vi "Scheduler.vi"(11 "Name (\"\" to Use UUID)":string) -> ()   [LabVIEW 2025]
uses:
  supports/Waypoint.ctl
  d7dd9159-89a2-4514-95bd-649e26e943bd.vi
  <vilib>/numeric/Random Number (Range) I64.vi
  e4e6d57c-e643-45f7-bca7-d28f1c2b9474.vi
  49f21eb9-f673-4fa8-8715-351f05abaff7.vi
  0d6ab66a-5149-4c79-b89e-f55ee53f3b39.vi
  3f08c095-eb42-4770-a6b1-2c55b3203edd.vi
  cd06cb13-84a1-4604-9614-019e20008b86.vi
  f0e5e5ea-bc13-4fd2-839c-8ba34e31ea16.vi
  <userlib>/_NEVSTOP/Communicable State Machine(CSM)/AdvanceAPI/CSM - Revert Arguments-Safe String.vi
  <userlib>/_NEVSTOP/Communicable State Machine(CSM)/AdvanceAPI/CSM - Make String Arguments Safe.vi
  <userlib>/_NEVSTOP/Communicable State Machine(CSM)/AdvanceAPI/CSM - Break Down Multiple States String.vi
  <userlib>/_NEVSTOP/Communicable State Machine(CSM)/AdvanceAPI/CSM - Compact Multiple States.vi
  <vilib>/numeric/sub_Random U32.vi
  <userlib>/_NEVSTOP/Communicable State Machine(CSM)/AdvanceAPI/CSM - Keywords.vi
  <userlib>/_NEVSTOP/Communicable State Machine(CSM)/_Shared/Trim Single-line Text.vi
  <userlib>/_NEVSTOP/Communicable State Machine(CSM)/addons/MassData-Parameter/_support/FGV-MassData(lvlibp).vi
  <userlib>/_NEVSTOP/Communicable State Machine(CSM)/_Polymophic/Build Status Broadcast Message.vi
  <userlib>/_NEVSTOP/Communicable State Machine(CSM)/_Polymophic/Build Synchronous Message with Arguments.vi
  <userlib>/_NEVSTOP/Communicable State Machine(CSM)/Communicable State Machine.lvlib
panel:
  out "Error Occurred":errorcluster
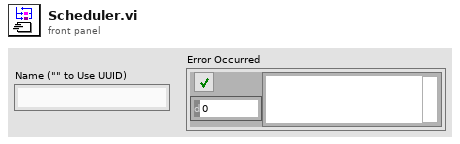
[diagram p1: front panel]
types:
  T1 = enum32{"Invalid", "Standard", "Closed", "Hidden", "Minimized", "Maximized"}
  T2 = enum32{"invalid app kind", "Development System", "Run Time System", "Student Edition", "Embedded LabVIEW", "Evaluation", "Custom"}
  T3 = typedef "Waypoint.ctl" = cluster{"x":i32, "y":i32}
  T4 = typedef "Communicable State Machine.lvlib/_CSM_Response Source Message.ctl" = cluster{"‘State":string, "’Arguments":string, "’Error":errorcluster}
  T5 = cluster{"Current VI Reference":refnum<vi>, "Close Panel on Exit?":bool}
  T6 = cluster{"Core":cluster{"Current VI Reference":refnum<vi>, "Close Panel on Exit?":bool}, "Level":i32, "Path":T3[], "Waypoint":T3, "Strike":i32, "Strikeout":i32, "Trial Count":i32}
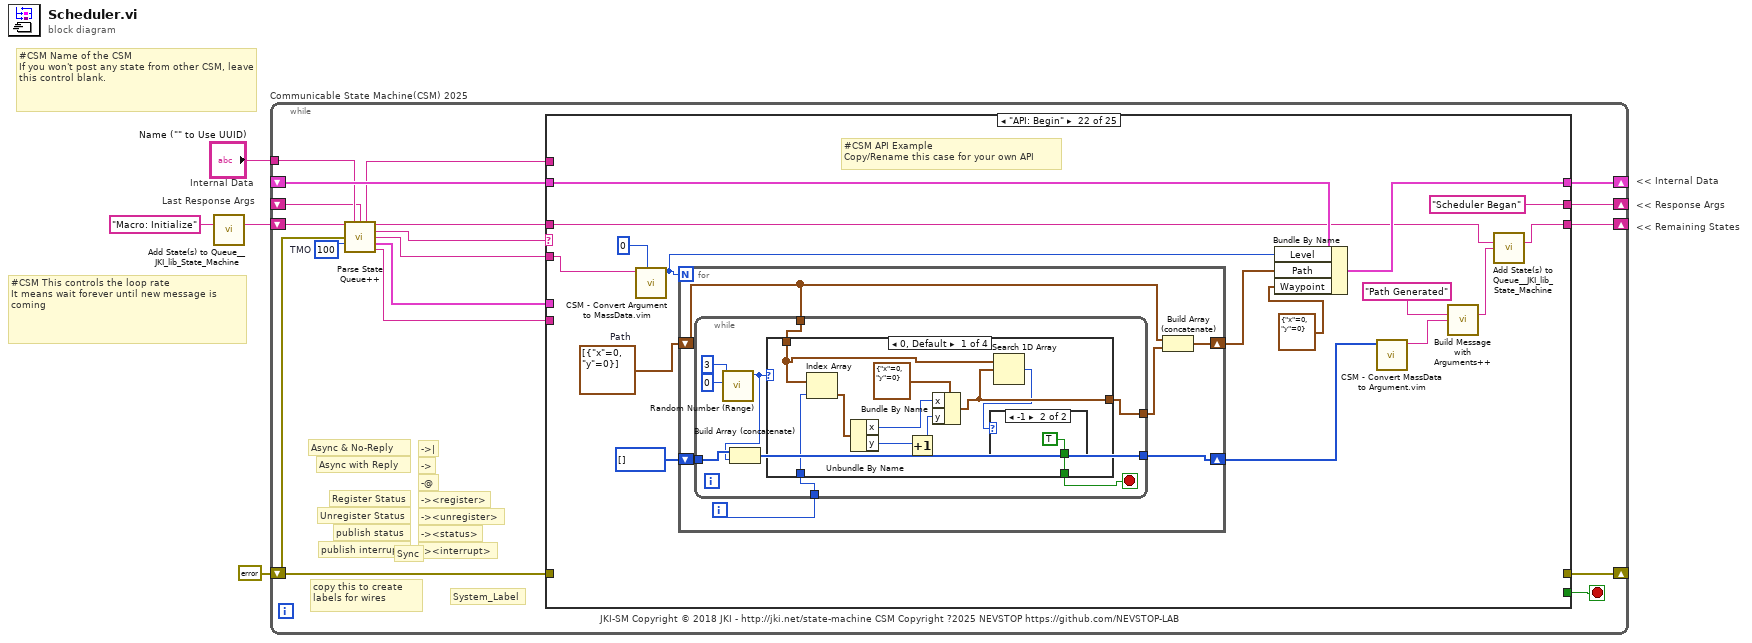
[diagram p0: block diagram]
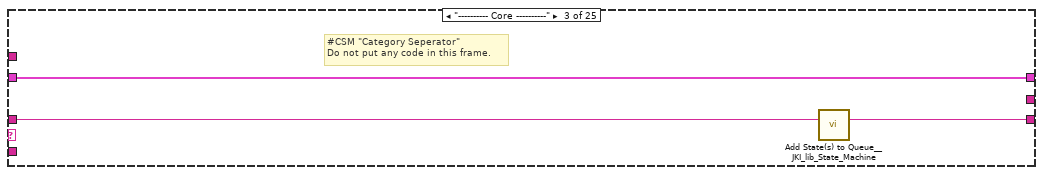
[diagram p4: hidden frame]
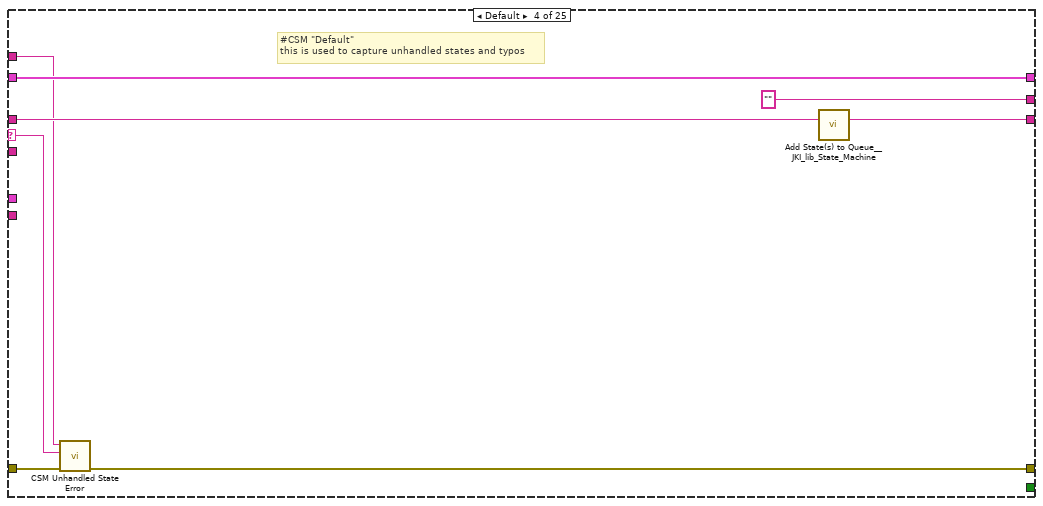
[diagram p5: hidden frame]
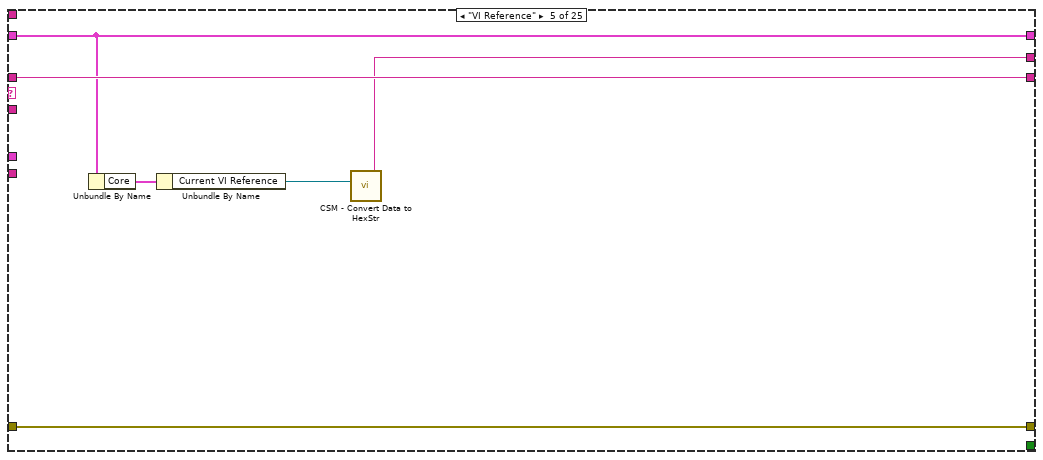
[diagram p6: hidden frame]
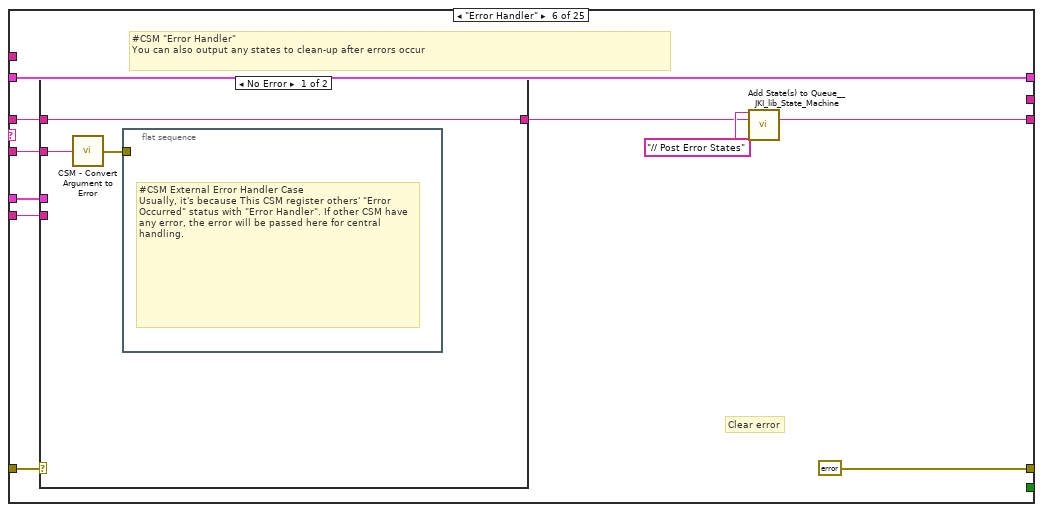
[diagram p7: hidden frame]
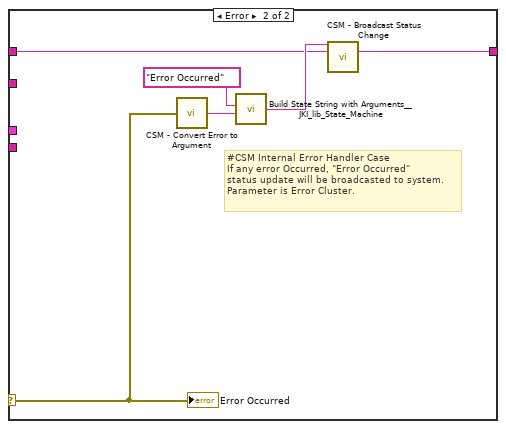
[diagram p8: hidden frame]
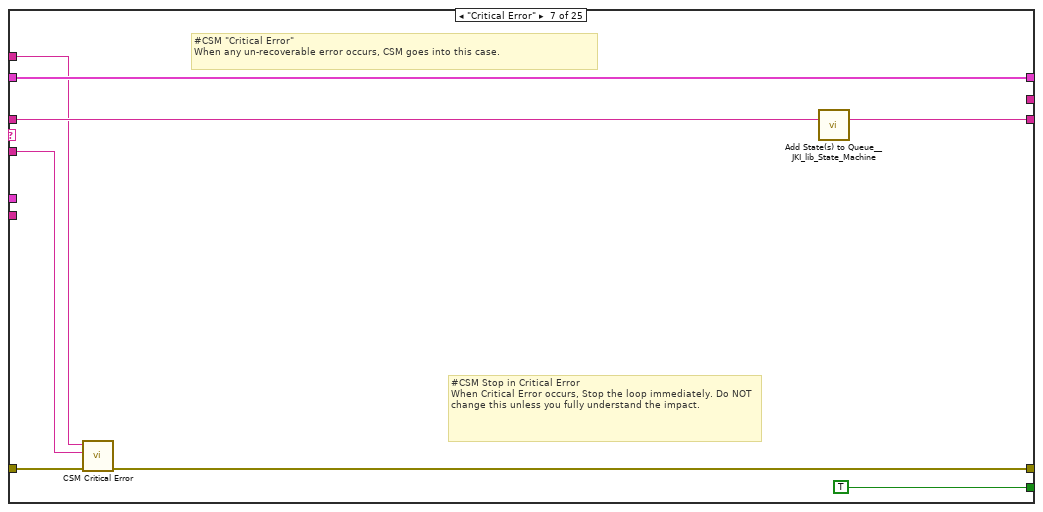
[diagram p9: hidden frame]
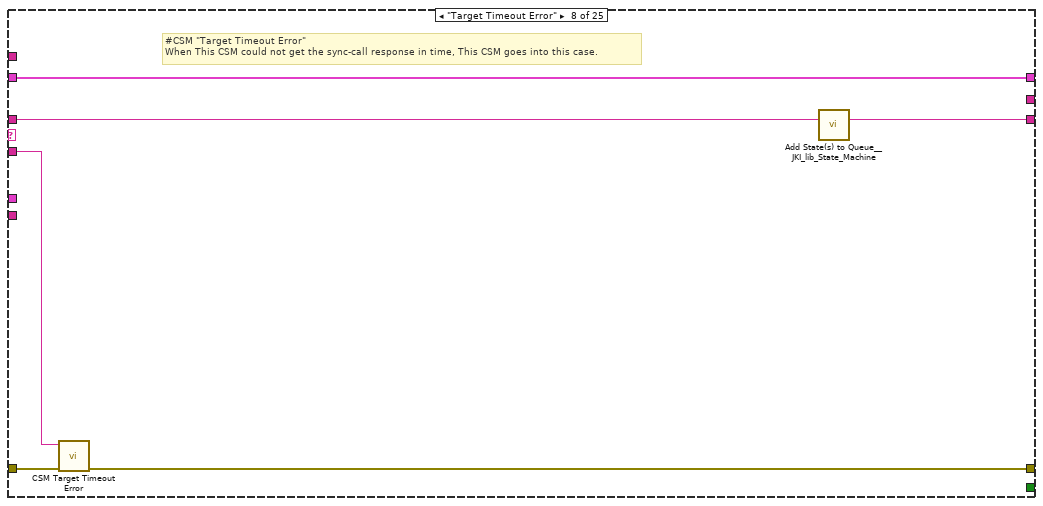
[diagram p10: hidden frame]
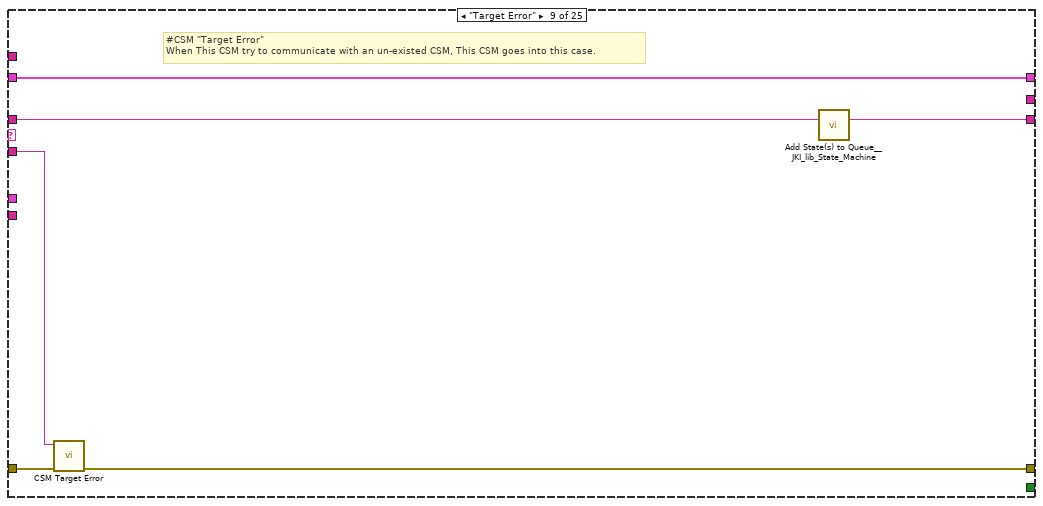
[diagram p11: hidden frame]
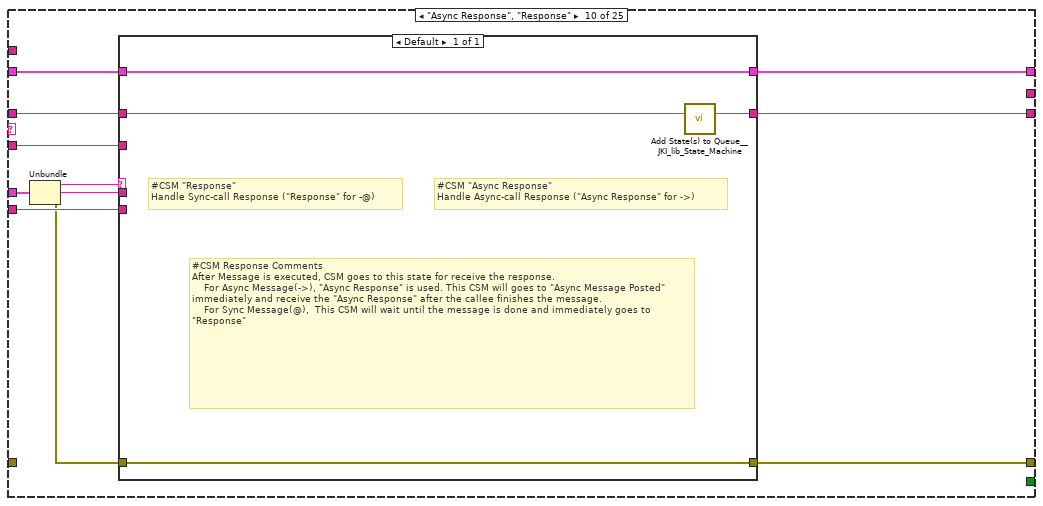
[diagram p12: hidden frame]
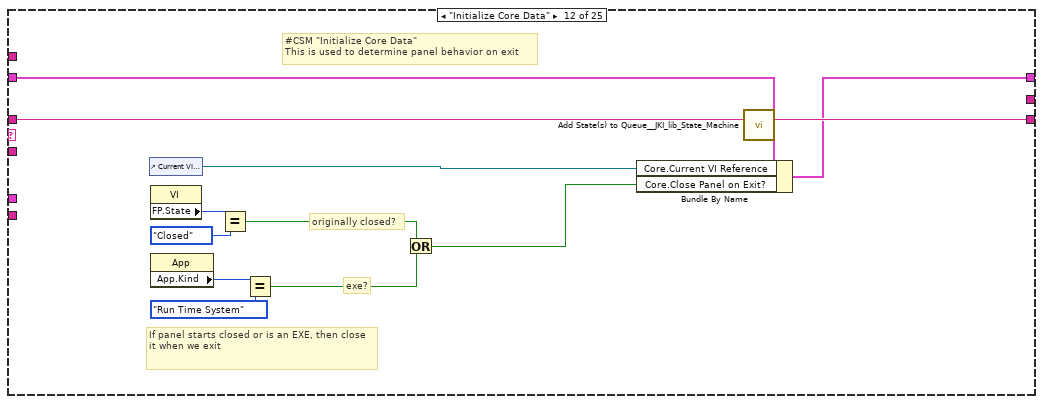
[diagram p14: hidden frame]
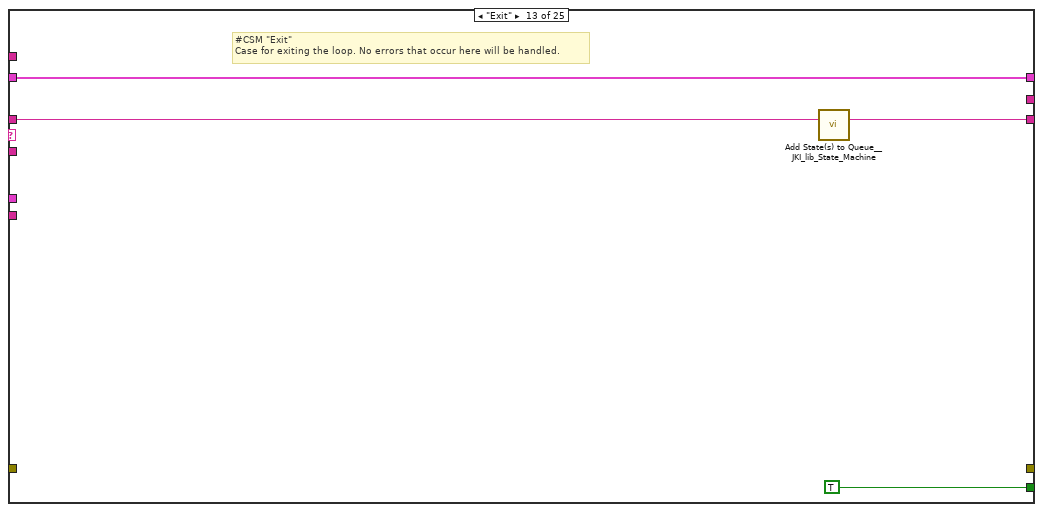
[diagram p15: hidden frame]
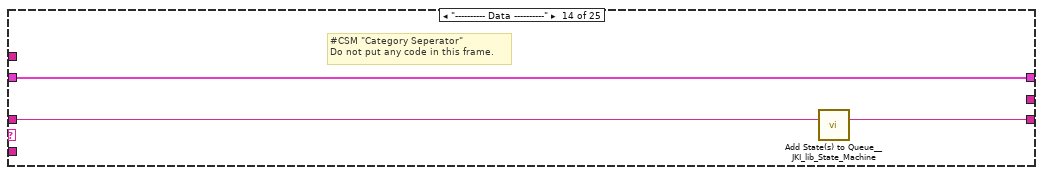
[diagram p16: hidden frame]
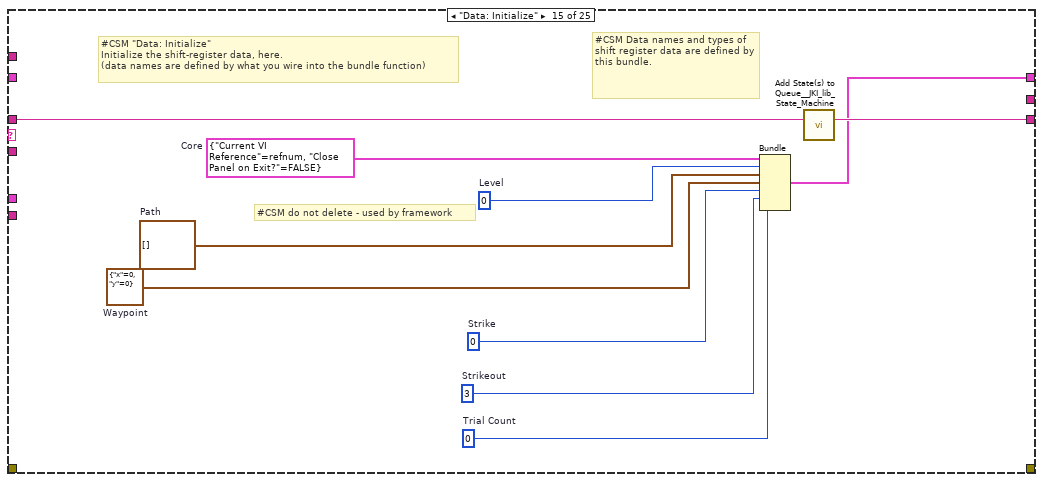
[diagram p17: hidden frame]
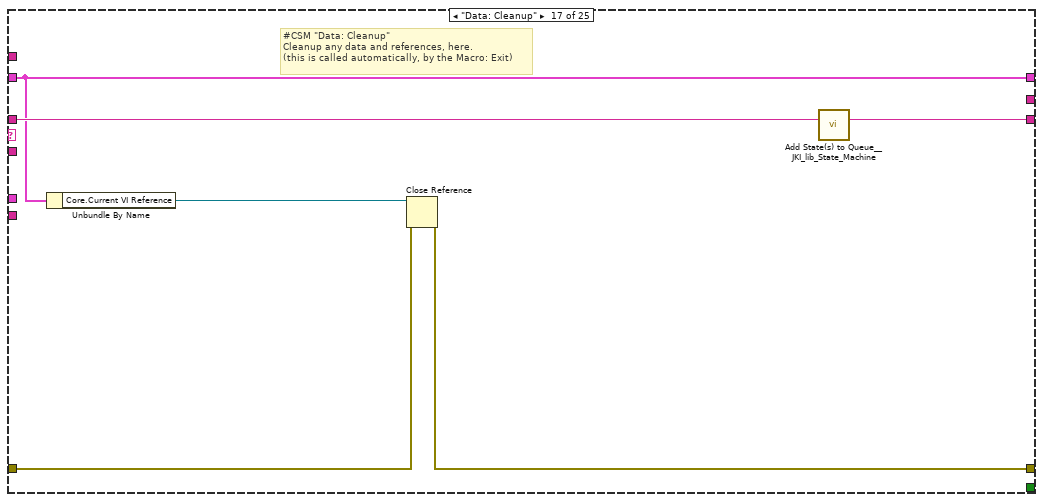
[diagram p19: hidden frame]
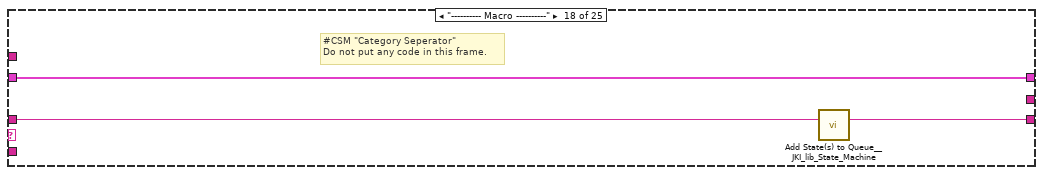
[diagram p20: hidden frame]
diagram:
  # "Last Response Args"
  # "Internal Data"
  # "#CSM Name of the CSM\nIf you won't post any state from other CSM, leave this control blank."
  # "#CSM This controls the loop rate\nIt means wait forever until new message is coming"
  # "<< Internal Data"
  # "<< Response Args"
  # "<< Remaining States"
  n1 = call <vilib>:"Add State(s) to Queue__JKI_lib_State_Machine.vi"("State(s) in (\"\")"="Macro: Initialize" ("Init State(\"Macro: Initialize\")")) -> ("States Out"=w1:string)  [unwired: 14 in]
  n2 = while "Communicable State Machine(CSM) 2025" {
    shift-right: [w16] -> _
    shift-left: _ -> [w15]
    shift-right: [w19] -> _
    shift-left: errorcluster {"status"=FALSE, "code"=0, "source"=""} ("error out") -> [w5]
    shift-right: [w18] -> _
    shift-left: w1 -> [w20]
    tunnel: "Name (\"\" to Use UUID)" -> [w12]
    shift-right: [w13] -> _
    shift-left: _ -> [w7]
    stop <- w17 stop-if-true
    w14 = 100  # TMO
    # "-><interrupt>"
    # "-><status>"
    # "-><unregister>"
    # "-><register>"
    # "-@"
    # "->"
    # "->|"
    # "publish interrupt"
    # "publish status"
    # "Unregister Status"
    # "Register Status"
    # "Sync"
    # "Async with Reply"
    # "Async & No-Reply"
    # "JKI-SM Copyright © 2018 JKI - http://jki.net/state-machine CSM Copyright ?2025 NEVSTOP https://github.com/NEVSTOP-LAB"
    # "copy this to create labels for wires"
    # "System_Label"
    n3 = call <userlib>:"Parse State Queue++.vi"("State Queue"=w20, "Name (\"\" to Use UUID)"=w12, "Response Arguments"=w7, "Previous Error"=w5, "Dequeue (1 ms)"=w14) -> ("Name Used"=w6:string, "Remaining States"=w21:string, "Current State"=w8:string, "Arguments"=w9:string, "Additional Information"=w10:T4, "Source CSM"=w11:string)  [unwired: 5 in]
    n4 = case shown="\"API: Begin\"" w8 {
      selector: w8 -> [_ _ _ w32 _ _ _ _ _ _ _ _ _ _ _ _ _ _ _ _ _ _ _ _ _]
      tunnel: w21 -> [w22 w25 w28 w36 w41 w46 w69 w75 w81 w91 w98 w110 w114 w117 w127 w129 w135 w138 w142 w148 w150 w158 w244 w371 w390]
      tunnel: w9 -> [_ _ _ _ _ w45 w65 w72 w78 w85 _ _ _ _ _ _ _ _ _ _ _ w164 w246 _ _]
      tunnel: w15 -> [w23 w24 w26 w34 w40 w51 w67 w73 w79 w89 w97 w104 w112 w115 _ w128 w130 w136 w140 w146 w149 w166 w245 w369 w383]
      tunnel: [_ _ _ w29 w42 errorcluster {"status"=FALSE, "code"=0, "source"=""} ("error out") w62 w70 w76 w92 _ _ _ _ _ _ w131 _ _ _ _ _ _ _ _] -> w19
      tunnel: w5 -> [_ _ _ w30 w42 w49 w63 w71 w77 _ _ _ _ _ _ _ w132 _ _ _ _ _ _ _ _]
      tunnel: [w22 w25 w27 w35 w41 w47 w68 w74 w80 w90 w98 w109 w113 w116 w126 w129 w134 w137 w141 w147 w150 w157 w240 w370 w389] -> w18
      tunnel: [_ _ _ _ _ _ TRUE _ _ _ _ _ TRUE _ _ _ _ _ _ _ _ _ _ _ _] -> w17
      tunnel: [w23 w24 w26 w34 w40 w51 w67 w73 w79 w88 w97 w108 w112 w115 w125 w128 w130 w136 w140 w146 w149 w165 w232 w369 w387] -> w16
      tunnel: w11 -> [_ _ _ _ _ w44 _ _ _ w86 _ _ _ _ _ _ _ _ _ _ _ _ _ _ _]
      tunnel: w10 -> [_ _ _ _ _ w43 _ _ _ w87 _ _ _ _ _ _ _ _ _ _ _ _ _ _ _]
      tunnel: [_ _ _ "" w37 _ _ _ _ _ _ _ _ _ _ _ _ _ _ _ _ "Scheduler Began" ("HEX String (0-9,A-F)") _ _ _] -> w13
      tunnel: w6 -> [_ _ _ w31 _ _ w64 _ _ _ _ _ _ _ _ _ _ _ _ _ _ _ _ _ _]
      frame "", "Idle" {
        # "#CSM \"Idle/Event Handler\"\nexecutes when the state queue is empty"
      }
      frame "CSM Documentation" {
        # "#CSM State Syntax\n\n// Comment line, all text to the right of “//” will be ignored\n// Local Message Example\nDoSth: DoA >> Arguments\n\n// Sync Call Example\nAPI: xxxx >> Arguments -@ TargetModule\n\n// Async Call Example\nAPI: xxxx >> Arguments -> TargetModule\n\n// Async Call without Reply Example\nAPI: xxxx >> Arguments ->| TargetModule\n\n// Broadcast normal status:\nStatus >> StatusArguments  -><status>\n\n// Broadcast Interrupt status:\nInterrupt >> StatusArguments  -><interrupt>\n\n// Register Source Module's status to Handler Module\nStatus@Source Module >> Handler Module@Handler Module -><register>\n\n// Unegister Source Module's status\nStatus@Source Module >> Handler Module -><unregister>"
        # "#CSM README FIRST\n\nCommunicable State Machine(CSM) is a LabVIEW application framework that builds upon JKI State Machine(JKISM). It follows the pattern of JKISM and extends the keywords to describe message communication between modules, including concepts such as Sync-Message, Async-Message, Subscription/Unsubscription of status - essential elements for creating reusable code modules. For more information, please visit the CSM wiki: https://nevstop-lab.github.io/CSM-Wiki/\n\nFor instructions on JKI State Machine, visit: \n    http://jki.net/state-machine/\nFor information about CSM, visit: \n    https://github.com/NEVSTOP-LAB"
        # "#CSM \"Documentation\"\nCase for holding CSM Documenation"
      }
      frame "---------- Core ----------" {
        # "#CSM \"Category Seperator\"\nDo not put any code in this frame."
        n5 = call <vilib>:"Add State(s) to Queue__JKI_lib_State_Machine.vi"("State(s) in (\"\")"=w28) -> ("States Out"=w27:string)  [unwired: 14 in]
      }
      frame Default {
        # "#CSM \"Default\"\nthis is used to capture unhandled states and typos"
        n6 = call <userlib>:"CSM Unhandled State Error.vi"("error in (no error)"=w30, "Undefined State"=w32, "CSM Name"=w31) -> ("error out"=w29:errorcluster)  [unwired: 8 in]
        n7 = call <vilib>:"Add State(s) to Queue__JKI_lib_State_Machine.vi"("State(s) in (\"\")"=w36) -> ("States Out"=w35:string)  [unwired: 14 in]
      }
      frame "VI Reference" {
        n8 = Unbundle By Name(w40) -> ("Core"=w39:T5)
        n9 = Unbundle By Name(w39) -> ("Current VI Reference"=w38:refnum<vi>)
        n10 = call <userlib>:"CSM - Convert Data to HexStr.vi"("Variant"=w38) -> ("HEX String (0-9,A-F)"=w37:string)  [unwired: 8 in]
      }
      frame "Error Handler" {
        # "#CSM \"Error Handler\"\nYou can also output any states to clean-up after errors occur"
        # "Clear error"
        n11 = case shown="No Error" w49 {
          selector: w49 -> [_ w56]
          tunnel: [w55 w58] -> w48
          tunnel: w46 -> [w55 w57]
          tunnel: w45 -> [w54 _]
          tunnel: w44 -> [_ _]
          tunnel: w43 -> [_ _]
          frame No Error {
            n12 = call <userlib>:"CSM - Convert Argument to Error.vi"("Argument"=w54) -> ("Error"=w53:errorcluster)  [unwired: 4 in]
            n13 = flat-sequence {
              tunnel: w53 -> [_]
              frame #0 {
                # "#CSM External Error Handler Case\nUsually, it's because This CSM register others' \"Error Occurred\" status with \"Error Handler\". If other CSM have any error, the error will be passed here for central handling."
              }
            }
          }
          frame Error {
            # "#CSM Internal Error Handler Case \nIf any error Occurred, \"Error Occurred\" \nstatus update will be broadcasted to system.\nParameter is Error Cluster."
            n14 = call <userlib>:"CSM - Convert Error to Argument.vi"("Error"=w56) -> ("Argument"=w60:string)  [unwired: 4 in]
            n15 = call <vilib>:"Build State String with Arguments__JKI_lib_State_Machine.vi"("Arguments (\"\")"=w60, "State"="Error Occurred" ("Status with Arguments")) -> ("State with Arguments"=w59:string)  [unwired: 4 in]
            n16 = call <userlib>:"CSM - Broadcast Status Change.vi"("Status With Arguments"=w59, "State Queue"=w57) -> ("Remaining States"=w58:string)  [unwired: 13 in]
            "Error Occurred" <- w56
          }
        }
        n17 = call <vilib>:"Add State(s) to Queue__JKI_lib_State_Machine.vi"("State(s) in Front (\"\")"="// Post Error States", "State(s) in (\"\")"=w48) -> ("States Out"=w47:string)  [unwired: 13 in]
      }
      frame "Critical Error" {
        # "#CSM \"Critical Error\"\nWhen any un-recoverable error occurs, CSM goes into this case."
        # "#CSM Stop in Critical Error\nWhen Critical Error occurs, Stop the loop immediately. Do NOT change this unless you fully understand the impact."
        n18 = call <userlib>:"CSM Critical Error.vi"("error in (no error)"=w63, "Arugments (As Reason)"=w65, "CSM Name"=w64) -> ("error out"=w62:errorcluster)  [unwired: 8 in]
        n19 = call <vilib>:"Add State(s) to Queue__JKI_lib_State_Machine.vi"("State(s) in (\"\")"=w69) -> ("States Out"=w68:string)  [unwired: 14 in]
      }
      frame "Target Timeout Error" {
        # "#CSM \"Target Timeout Error\"\nWhen This CSM could not get the sync-call response in time, This CSM goes into this case."
        n20 = call <userlib>:"CSM Target Timeout Error.vi"("error in (no error)"=w71, "Arguments (As CSM Name)"=w72) -> ("error out"=w70:errorcluster)  [unwired: 9 in]
        n21 = call <vilib>:"Add State(s) to Queue__JKI_lib_State_Machine.vi"("State(s) in (\"\")"=w75) -> ("States Out"=w74:string)  [unwired: 14 in]
      }
      frame "Target Error" {
        # "#CSM \"Target Error\"\nWhen This CSM try to communicate with an un-existed CSM, This CSM goes into this case."
        n22 = call <userlib>:"CSM Target Error.vi"("error in (no error)"=w77, "Arguments (As CSM Name)"=w78) -> ("error out"=w76:errorcluster)  [unwired: 9 in]
        n23 = call <vilib>:"Add State(s) to Queue__JKI_lib_State_Machine.vi"("State(s) in (\"\")"=w81) -> ("States Out"=w80:string)  [unwired: 14 in]
      }
      frame "Async Response", "Response" {
        n24 = Unbundle(w87) -> ("‘State"=w84:string, "’Arguments"=w83:string, "’Error"=w82:errorcluster)
        n25 = case shown="Default" w84 {
          tunnel: [w93] -> w90
          tunnel: w91 -> [w94]
          tunnel: [w96] -> w88
          tunnel: w89 -> [w96]
          tunnel: [w95] -> w92
          tunnel: w82 -> [w95]
          tunnel: w86 -> [_]
          tunnel: w85 -> [_]
          tunnel: w83 -> [_]
          frame Default {
            # "#CSM \"Async Response\"\nHandle Async-call Response (\"Async Response\" for ->)"
            # "#CSM \"Response\"\nHandle Sync-call Response (\"Response\" for -@)"
            # "#CSM Response Comments\nAfter Message is executed, CSM goes to this state for receive the response.\n    For Async Message(->), \"Async Response\" is used. This CSM will goes to \"Async Message Posted\" immediately and receive the \"Async Response\" after the callee finishes the message.\n    For Sync Message(@),  This CSM will wait until the message is done and immediately goes to \"Response\""
            n26 = call <vilib>:"Add State(s) to Queue__JKI_lib_State_Machine.vi"("State(s) in (\"\")"=w94) -> ("States Out"=w93:string)  [unwired: 14 in]
          }
        }
      }
      frame "Async Message Posted" {
        # "#CSM \"Async Message Posted\"\nAfter Async Message is posted (-> or ->| ), CSM goes to this state for post-action.\nYou can use Argument - State to tell which Async Message is called."
      }
      frame "Initialize Core Data" {
        # "#CSM \"Initialize Core Data\"\nThis is used to determine panel behavior on exit"
        # "originally closed?"
        # "exe?"
        # "If panel starts closed or is an EXE, then close it when we exit"
        n27 = control-ref of="Current VI Reference"() -> (w102:refnum<vi>)
        n28 = property class="VI"() -> ("FP.State"=w101:T1)  [unwired: 2 in, 2 out]
        n29 = property class="App"() -> ("App.Kind"=w107:T2)  [unwired: 2 in, 2 out]
        n30 = Equal?(x=w101, y=T1."Closed" ("Front Panel Window:State")) -> (x = y?=w99:bool)
        n31 = Equal?(x=w107, y=T2."Run Time System" ("Application:Kind")) -> (x = y?=w105:bool)
        n32 = Or(x=w99, y=w105) -> (x .or. y?=w103:bool)
        n33 = Bundle By Name(cluster=w104, "Core.Current VI Reference"=w102, "Core.Close Panel on Exit?"=w103) -> (w108:T6)
        n34 = call <vilib>:"Add State(s) to Queue__JKI_lib_State_Machine.vi"("State(s) in (\"\")"=w110) -> ("States Out"=w109:string)  [unwired: 14 in]
      }
      frame "Exit" {
        # "#CSM \"Exit\"\nCase for exiting the loop. No errors that occur here will be handled."
        n35 = call <vilib>:"Add State(s) to Queue__JKI_lib_State_Machine.vi"("State(s) in (\"\")"=w114) -> ("States Out"=w113:string)  [unwired: 14 in]
      }
      frame "---------- Data ----------" {
        # "#CSM \"Category Seperator\"\nDo not put any code in this frame."
        n36 = call <vilib>:"Add State(s) to Queue__JKI_lib_State_Machine.vi"("State(s) in (\"\")"=w117) -> ("States Out"=w116:string)  [unwired: 14 in]
      }
      frame "Data: Initialize" {
        w118 = 0  # Trial Count
        w119 = 3  # Strikeout
        w120 = 0  # Strike
        w121 = T3 {"x"=0, "y"=0}  # Waypoint
        w122 = T3[] []  # Path
        w123 = 0  # Level
        w124 = T5 {"Current VI Reference"=refnum, "Close Panel on Exit?"=FALSE}  # Core
        # "#CSM \"Data: Initialize\"\nInitialize the shift-register data, here.\n(data names are defined by what you wire into the bundle function)"
        # "#CSM do not delete - used by framework"
        # "#CSM Data names and types of shift register data are defined by this bundle."
        n37 = Bundle("Core"=w124, "Level"=w123, "Path"=w122, "Waypoint"=w121, "Strike"=w120, "Strikeout"=w119, "Trial Count"=w118) -> (w125:T6)  [unwired: 1 in]
        n38 = call <vilib>:"Add State(s) to Queue__JKI_lib_State_Machine.vi"("State(s) in (\"\")"=w127) -> ("States Out"=w126:string)  [unwired: 14 in]
      }
      frame "Data: Update Indicators" {
      }
      frame "Data: Cleanup" {
        # "#CSM \"Data: Cleanup\"\nCleanup any data and references, here.\n(this is called automatically, by the Macro: Exit)"
        n39 = Unbundle By Name(w130) -> ("Core.Current VI Reference"=w133:refnum<vi>)
        n40 = Close Reference(reference=w133, error in (no error)=w132) -> (error out=w131:errorcluster)
        n41 = call <vilib>:"Add State(s) to Queue__JKI_lib_State_Machine.vi"("State(s) in (\"\")"=w135) -> ("States Out"=w134:string)  [unwired: 14 in]
      }
      frame "---------- Macro ----------" {
        # "#CSM \"Category Seperator\"\nDo not put any code in this frame."
        n42 = call <vilib>:"Add State(s) to Queue__JKI_lib_State_Machine.vi"("State(s) in (\"\")"=w138) -> ("States Out"=w137:string)  [unwired: 14 in]
      }
      frame "Macro: Initialize" {
        # "#CSM \"Macro: Initialize\"\nInitialization Macro (This is called once, when the VI starts)"
        n43 = call <vilib>:"Add State(s) to Queue__JKI_lib_State_Machine.vi"("State(s) in Front (\"\")"="Initialize Core Data\nData: Initialize\nData: Update Indicators", "State(s) in (\"\")"=w142) -> ("States Out"=w141:string)  [unwired: 13 in]
      }
      frame "Macro: Exit" {
        # "#CSM \"Macro: Exit\"\nExit Macro (This is called once, when the VI exits)"
        n44 = call <vilib>:"Add State(s) to Queue__JKI_lib_State_Machine.vi"("State(s) in Front (\"\")"="//Exit Sub-Modules ", "State(s) at Back (\"\")"="Data: Cleanup\nExit") -> ("States Out"=w144:string)  [unwired: 13 in]
        n45 = call <vilib>:"Add State(s) to Queue__JKI_lib_State_Machine.vi"("State(s) in Front (\"\")"=w144, "State(s) in (\"\")"=w148) -> ("States Out"=w147:string)  [unwired: 13 in]
      }
      frame "---------- API ----------" {
        # "#CSM \"Category Seperator\"\nDo not put any code in this frame."
      }
      frame "API: Begin" {
        w162 = T3[] [{"x"=0, "y"=0}]  # Path
        # "#CSM API Example\nCopy/Rename this case for your own API"
        n46 = call "CSM - Convert Argument to MassData.vim"("Type"=0, "MassData Argument"=w164) -> ("Data"=w160:i32)  [unwired: 6 in, 1 out]
        n47 = for {
          N: w160 -> [_]
          shift-right: [w172] -> w154
          shift-left: w162 -> [w171]
          shift-right: [w167] -> w151
          shift-left: i64[] [] ("appended array") -> [w168]
          i -> [w170]
          n48 = while {
            tunnel: w171 -> [w179]
            tunnel: w170 -> [w178]
            tunnel: [w177] -> w169
            tunnel: w168 -> [w175]
            tunnel: [w174] -> w167
            stop <- w176 stop-if-true
            n49 = call-poly <vilib>:"Random Number (Range).vi"("lower bound (-100)"=i64 0, "upper bound (100)"=i64 3) -> ("number"=w173:i64)  [unwired: 9 in]
            n50 = Build Array (concatenate)(w175, w173) -> (w174:i64[])
            n51 = case shown="0, Default" w173 {
              tunnel: w179 -> [w188 w200 w211 w221]
              tunnel: w178 -> [w191 w203 w215 w227]
              tunnel: [w187 w199 w210 w220] -> w177
              tunnel: [w185 w197 w208 w218] -> w176
              frame 0, Default {
                n52 = Index Array(array=w188, index=w191) -> (element=w190:T3)
                n53 = Unbundle By Name(w190) -> ("x"=w184:i32, "y"=w183:i32)
                n54 = Increment(x=w183) -> (x+1=w182:i32)
                n55 = Bundle By Name(cluster=T3 {"x"=0, "y"=0} ("Waypoint"), "x"=w184, "y"=w182) -> (w187:T3)
                n56 = Search 1D Array(1D array=w188, element=w187) -> (index of element=w186:i32)  [unwired: 1 in]
                n57 = case shown="-1" w186 {
                  tunnel: [FALSE TRUE] -> w185
                  frame Default {
                  }
                  frame -1 {
                  }
                }
              }
              frame 1 {
                n58 = Index Array(array=w200, index=w203) -> (element=w202:T3)
                n59 = Unbundle By Name(w202) -> ("x"=w196:i32, "y"=w195:i32)
                n60 = Decrement(x=w195) -> (x-1=w194:i32)
                n61 = Bundle By Name(cluster=T3 {"x"=0, "y"=0} ("Waypoint"), "x"=w196, "y"=w194) -> (w199:T3)
                n62 = Search 1D Array(1D array=w200, element=w199) -> (index of element=w198:i32)  [unwired: 1 in]
                n63 = case shown="-1" w198 {
                  tunnel: [FALSE TRUE] -> w197
                  frame Default {
                  }
                  frame -1 {
                  }
                }
              }
              frame 2 {
                n64 = Index Array(array=w211, index=w215) -> (element=w214:T3)
                n65 = Unbundle By Name(w214) -> ("x"=w207:i32, "y"=w212:i32)
                n66 = Decrement(x=w207) -> (x-1=w206:i32)
                n67 = Bundle By Name(cluster=T3 {"x"=0, "y"=0} ("Waypoint"), "x"=w206, "y"=w212) -> (w210:T3)
                n68 = Search 1D Array(1D array=w211, element=w210) -> (index of element=w209:i32)  [unwired: 1 in]
                n69 = case shown="-1" w209 {
                  tunnel: [FALSE TRUE] -> w208
                  frame Default {
                  }
                  frame -1 {
                  }
                }
              }
              frame 3 {
                n70 = Index Array(array=w221, index=w227) -> (element=w226:T3)
                n71 = Unbundle By Name(w226) -> ("x"=w225:i32, "y"=w222:i32)
                n72 = Increment(x=w225) -> (x+1=w224:i32)
                n73 = Bundle By Name(cluster=T3 {"x"=0, "y"=0} ("Waypoint"), "x"=w224, "y"=w222) -> (w220:T3)
                n74 = Search 1D Array(1D array=w221, element=w220) -> (index of element=w219:i32)  [unwired: 1 in]
                n75 = case shown="-1" w219 {
                  tunnel: [FALSE TRUE] -> w218
                  frame Default {
                  }
                  frame -1 {
                  }
                }
              }
            }
          }
          n76 = Build Array (concatenate)(w171, w169) -> (w172:T3[])
        }
        n77 = Bundle By Name(cluster=w166, "Level"=w160, "Path"=w154, "Waypoint"=T3 {"x"=0, "y"=0}) -> (w165:T6)
        n78 = call "CSM - Convert MassData to Argument.vim"("Data"=w151) -> ("MassData Argument"=w153:string)  [unwired: 7 in, 1 out]
        n79 = call-poly <userlib>:"Build Message with Arguments++.vi"("State With Arguments"="Path Generated", "Arguments (\"\")"=w153) -> ("CSM Message String"=w156:string)  [unwired: 13 in]
        n80 = call <vilib>:"Add State(s) to Queue__JKI_lib_State_Machine.vi"("State(s) in (\"\")"=w158, "State(s) at Back (\"\")"=w156) -> ("States Out"=w157:string)  [unwired: 13 in]
      }
      frame "API: Check Waypoint" {
        # "#CSM API Example\nCopy/Rename this case for your own API"
        n81 = case shown="\"Gate Up\"" w246 {
          tunnel: w245 -> [w264 w277 w303 w329 w355]
          tunnel: [w264 w267 w293 w320 w346] -> w233
          tunnel: "Gate Scheduled" -> [_ w272 w297 w317 w349]
          tunnel: [" \"Error Handler\" " w273 w296 w323 w343] -> w242
          frame Default {
          }
          frame "Gate Up" {
            n82 = Unbundle By Name(w277) -> ("Waypoint.x"=w278:i32, "Waypoint.y"=w280:i32)
            n83 = Increment(x=w280) -> (x+1=w279:i32)
            n84 = Bundle By Name(cluster=w277, "Waypoint.x"=w278, "Waypoint.y"=w279) -> (w268:T6)
            n85 = Unbundle By Name(w268) -> ("Path"=w275:T3[], "Waypoint"=w276:T3, "Level"=w269:i32, "Strike"=w266:i32)
            n86 = Search 1D Array(1D array=w275, element=w276) -> (index of element=w274:i32)  [unwired: 1 in]
            n87 = case shown="Default" w274 {
              selector: w274 -> [w284 _]
              tunnel: [w285 w290] -> w270
              tunnel: w269 -> [w283 _]
              tunnel: w266 -> [w281 w289]
              tunnel: [w281 w288] -> w265
              frame Default {
                n88 = Equal?(x=w284, y=w283) -> (x = y?=w282:bool)
                n89 = case shown="False" w282 {
                  tunnel: [w286 w287] -> w285
                  frame False {
                    w286 = bool[] [FALSE, FALSE, FALSE, FALSE]  # Gate Condition
                  }
                  frame True {
                    w287 = bool[] [TRUE, FALSE, TRUE, TRUE]  # Gate Condition
                  }
                }
              }
              frame -1 {
                w290 = bool[] [TRUE, FALSE, TRUE, TRUE]  # Gate Condition
                n90 = Increment(x=w289) -> (x+1=w288:i32)
              }
            }
            n91 = Bundle By Name(cluster=w268, "Strike"=w265) -> (w267:T6)
            n92 = call "CSM - Convert MassData to Argument.vim"("Data"=w270) -> ("MassData Argument"=w271:string)  [unwired: 7 in, 1 out]
            n93 = call-poly <userlib>:"Build Message with Arguments++.vi"("State With Arguments"=w272, "Arguments (\"\")"=w271) -> ("CSM Message String"=w273:string)  [unwired: 13 in]
          }
          frame "Gate Down" {
            n94 = Unbundle By Name(w303) -> ("Waypoint.x"=w305:i32, "Waypoint.y"=w306:i32)
            n95 = Decrement(x=w306) -> (x-1=w304:i32)
            n96 = Bundle By Name(cluster=w303, "Waypoint.x"=w305, "Waypoint.y"=w304) -> (w294:T6)
            n97 = Unbundle By Name(w294) -> ("Path"=w301:T3[], "Waypoint"=w302:T3, "Level"=w295:i32, "Strike"=w291:i32)
            n98 = Search 1D Array(1D array=w301, element=w302) -> (index of element=w300:i32)  [unwired: 1 in]
            n99 = case shown="Default" w300 {
              selector: w300 -> [w310 _]
              tunnel: [w308 w316] -> w299
              tunnel: w295 -> [w311 _]
              tunnel: [w307 w315] -> w292
              tunnel: w291 -> [w307 w314]
              frame Default {
                n100 = Equal?(x=w310, y=w311) -> (x = y?=w309:bool)
                n101 = case shown="False" w309 {
                  tunnel: [w312 w313] -> w308
                  frame False {
                    w312 = bool[] [FALSE, FALSE, FALSE, FALSE]  # Gate Condition
                  }
                  frame True {
                    w313 = bool[] [FALSE, TRUE, TRUE, TRUE]  # Gate Condition
                  }
                }
              }
              frame -1 {
                w316 = bool[] [FALSE, TRUE, TRUE, TRUE]  # Gate Condition
                n102 = Increment(x=w314) -> (x+1=w315:i32)
              }
            }
            n103 = Bundle By Name(cluster=w294, "Strike"=w292) -> (w293:T6)
            n104 = call "CSM - Convert MassData to Argument.vim"("Data"=w299) -> ("MassData Argument"=w298:string)  [unwired: 7 in, 1 out]
            n105 = call-poly <userlib>:"Build Message with Arguments++.vi"("State With Arguments"=w297, "Arguments (\"\")"=w298) -> ("CSM Message String"=w296:string)  [unwired: 13 in]
          }
          frame "Gate Left" {
            n106 = Unbundle By Name(w329) -> ("Waypoint.x"=w332:i32, "Waypoint.y"=w330:i32)
            n107 = Decrement(x=w332) -> (x-1=w331:i32)
            n108 = Bundle By Name(cluster=w329, "Waypoint.x"=w331, "Waypoint.y"=w330) -> (w321:T6)
            n109 = Unbundle By Name(w321) -> ("Path"=w327:T3[], "Waypoint"=w328:T3, "Level"=w322:i32, "Strike"=w319:i32)
            n110 = Search 1D Array(1D array=w327, element=w328) -> (index of element=w326:i32)  [unwired: 1 in]
            n111 = case shown="Default" w326 {
              selector: w326 -> [w336 _]
              tunnel: [w337 w342] -> w325
              tunnel: w322 -> [w334 _]
              tunnel: w319 -> [w333 w341]
              tunnel: [w333 w340] -> w318
              frame Default {
                n112 = Equal?(x=w336, y=w334) -> (x = y?=w335:bool)
                n113 = case shown="True" w335 {
                  tunnel: [w338 w339] -> w337
                  frame False {
                    w338 = bool[] [FALSE, FALSE, FALSE, FALSE]  # Gate Condition
                  }
                  frame True {
                    w339 = bool[] [TRUE, TRUE, TRUE, FALSE]  # Gate Condition
                  }
                }
              }
              frame -1 {
                w342 = bool[] [TRUE, TRUE, TRUE, FALSE]  # Gate Condition
                n114 = Increment(x=w341) -> (x+1=w340:i32)
              }
            }
            n115 = Bundle By Name(cluster=w321, "Strike"=w318) -> (w320:T6)
            n116 = call "CSM - Convert MassData to Argument.vim"("Data"=w325) -> ("MassData Argument"=w324:string)  [unwired: 7 in, 1 out]
            n117 = call-poly <userlib>:"Build Message with Arguments++.vi"("State With Arguments"=w317, "Arguments (\"\")"=w324) -> ("CSM Message String"=w323:string)  [unwired: 13 in]
          }
          frame "Gate Right" {
            n118 = Unbundle By Name(w355) -> ("Waypoint.x"=w358:i32, "Waypoint.y"=w356:i32)
            n119 = Increment(x=w358) -> (x+1=w357:i32)
            n120 = Bundle By Name(cluster=w355, "Waypoint.x"=w357, "Waypoint.y"=w356) -> (w347:T6)
            n121 = Unbundle By Name(w347) -> ("Path"=w353:T3[], "Waypoint"=w354:T3, "Level"=w348:i32, "Strike"=w344:i32)
            n122 = Search 1D Array(1D array=w353, element=w354) -> (index of element=w352:i32)  [unwired: 1 in]
            n123 = case shown="Default" w352 {
              selector: w352 -> [w361 _]
              tunnel: [w363 w368] -> w351
              tunnel: w348 -> [w360 _]
              tunnel: [w359 w367] -> w345
              tunnel: w344 -> [w359 w366]
              frame Default {
                n124 = Equal?(x=w361, y=w360) -> (x = y?=w362:bool)
                n125 = case shown="False" w362 {
                  tunnel: [w364 w365] -> w363
                  frame False {
                    w364 = bool[] [FALSE, FALSE, FALSE, FALSE]  # Gate Condition
                  }
                  frame True {
                    w365 = bool[] [TRUE, TRUE, FALSE, TRUE]  # Gate Condition
                  }
                }
              }
              frame -1 {
                w368 = bool[] [TRUE, TRUE, FALSE, TRUE]  # Gate Condition
                n126 = Increment(x=w366) -> (x+1=w367:i32)
              }
            }
            n127 = call "CSM - Convert MassData to Argument.vim"("Data"=w351) -> ("MassData Argument"=w350:string)  [unwired: 7 in, 1 out]
            n128 = Bundle By Name(cluster=w347, "Strike"=w345) -> (w346:T6)
            n129 = call-poly <userlib>:"Build Message with Arguments++.vi"("State With Arguments"=w349, "Arguments (\"\")"=w350) -> ("CSM Message String"=w343:string)  [unwired: 13 in]
          }
        }
        n130 = call <vilib>:"Add State(s) to Queue__JKI_lib_State_Machine.vi"("State(s) in (\"\")"=w244, "State(s) at Back (\"\")"=w242) -> ("States Out"=w241:string)  [unwired: 13 in]
        n131 = Unbundle By Name(w233) -> ("Trial Count"=w231:i32, "Path"=w238:T3[], "Waypoint"=w237:T3, "Level"=w239:i32, "Strike"=w235:i32, "Strikeout"=w234:i32)
        n132 = Equal?(x=w235, y=w234) -> (x = y?=w236:bool)
        n133 = case shown="False" w236 {
          tunnel: w241 -> [w251 w252]
          tunnel: [w250 w257] -> w240
          tunnel: w239 -> [_ w253]
          tunnel: w238 -> [_ w255]
          tunnel: w237 -> [_ w254]
          frame True {
            n134 = call-poly <userlib>:"Build Message with Arguments++.vi"("State With Arguments"="Macro: Exit", "Target Module (\"\")"="main" ("Target Module (\"\")")) -> ("CSM Message String"=w247:string)  [unwired: 13 in]
            n135 = call <vilib>:"Add State(s) to Queue__JKI_lib_State_Machine.vi"("State(s) in (\"\")"=w251, "State(s) at Back (\"\")"=w247) -> ("States Out"=w250:string)  [unwired: 13 in]
          }
          frame False {
            n136 = Search 1D Array(1D array=w255, element=w254) -> (index of element=w256:i32)  [unwired: 1 in]
            n137 = Equal?(x=w256, y=w253) -> (x = y?=w258:bool)
            n138 = case shown="True" w258 {
              tunnel: [w259 w262] -> w257
              tunnel: w252 -> [w259 w260]
              frame False {
              }
              frame True {
                n139 = call <vilib>:"Add State(s) to Queue__JKI_lib_State_Machine.vi"("State(s) in (\"\")"=w260, "State(s) at Back (\"\")"="Action: Start New Game" ("State(s) at Back (\"\")")) -> ("States Out"=w262:string)  [unwired: 13 in]
              }
            }
          }
        }
        n140 = Increment(x=w231) -> (x+1=w230:i32)
        n141 = Build Array(w237) -> ()  [unwired: 1 out]
        n142 = Bundle By Name(cluster=w233, "Trial Count"=w230) -> (w232:T6)
      }
      frame "---------- Action ----------" {
        # "#CSM \"Category Seperator\"\nDo not put any code in this frame."
        n143 = call <vilib>:"Add State(s) to Queue__JKI_lib_State_Machine.vi"("State(s) in (\"\")"=w371) -> ("States Out"=w370:string)  [unwired: 14 in]
      }
      frame "Action: Start New Game" {
        w385 = 0 ("Strike")
        # "#CSM \"Internal State\"\nThis category is used for holding internal states"
        n144 = Unbundle By Name(w383) -> ("Level"=w377:i32, "Trial Count"=w382:i32)
        n145 = Subtract(x=w377, y=w382) -> (x-y=w381:i32)
        n146 = Increment(x=w381) -> (x+1=w380:i32)
        n147 = In Range and Coerce(upper limit=w377, x=w380, lower limit=0) -> (coerced(x)=w378:i32)  [unwired: 1 out]
        n148 = call "CSM - Convert MassData to Argument.vim"("Data"=w378) -> ("MassData Argument"=w384:string)  [unwired: 7 in, 1 out]
        n149 = call-poly <userlib>:"Build Message with Arguments++.vi"("State With Arguments"="API: Level Up", "Target Module (\"\")"="main" ("Target Module (\"\")")) -> ("CSM Message String"=w372:string)  [unwired: 13 in]
        n150 = call-poly <userlib>:"Build Message with Arguments++.vi"("State With Arguments"="Macro: Game Start", "Arguments (\"\")"=w384, "Target Module (\"\")"="main" ("Target Module (\"\")")) -> ("CSM Message String"=w375:string)  [unwired: 12 in]
        n151 = call <vilib>:"Add State(s) to Queue__JKI_lib_State_Machine.vi"("State(s) in Front (\"\")"=w372, "State(s) in (\"\")"=w390, "State(s) at Back (\"\")"=w375) -> ("States Out"=w389:string)  [unwired: 12 in]
        n152 = Bundle By Name(cluster=w383, "Waypoint"=T3 {"x"=0, "y"=0}, "Strike"=w385, "Trial Count"=w385) -> (w387:T6)
      }
    }
  }
